vi "3DmenuHandler.vi"(4 "nearClip":sgl, 5 "RawDataFile":path, 6 "farClip":sgl, 7 "FoV":sgl, 10 "ItemTag":string, 11 "3DpicRef":refnum<vi>) -> (0 "error out":errorcluster)   [LabVIEW 2022 SP3]
uses:
  <vilib>/Utility/miscctls.llb/LV3DPointTypeDef.ctl
  <vilib>/Utility/miscctls.llb/LVRectTypeDef.ctl
  <vilib>/Analysis/Matrix/Datatypes/RealMatrix.ctl
  <vilib>/Analysis/baseanly.llb/Matrix Type of Inverse Matrix.ctl
  <vilib>/Analysis/baseanly.llb/Real A x B.vi
  Anemometry/Anemometry Sub Vis/Data_plotting_vis/Results_plotter_Global.vi
  <vilib>/Platform/browser.llb/Open URL in Default Browser (path).vi
  <vilib>/Analysis/baseanly.llb/Real Inverse Matrix.vi
  <vilib>/picture/3D Picture Control/NI_3D Picture Control.lvlib
  <vilib>/Analysis/NI_AALBase.lvlib
  <vilib>/Analysis/Matrix/NI_Matrix.lvlib
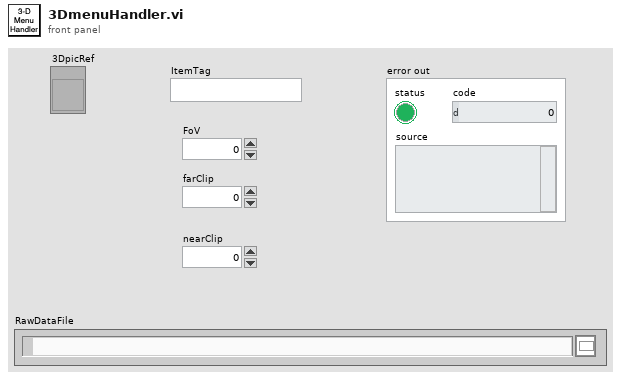
[diagram p1: front panel]
types:
  T1 = enum16{"None", "Spherical", "Flying", "Oriented"}
  T2 = typedef "LV3DPointTypeDef.ctl" = cluster{"X":sgl, "Y":sgl, "Z":sgl}
  T3 = typedef "NI_AALBase.lvlib/Matrix Type of Inverse Matrix.ctl" = enum32{"General", "Positive Definite", "Lower Triangular", "Upper Triangular"}
  T4 = typedef "NI_Matrix.lvlib/RealMatrix.ctl" = dbl[][]
  T5 = enum16{"Open", "Minimized", "Maximized", "Hidden"}
  T6 = typedef "LVRectTypeDef.ctl" = cluster{"Left":i16, "Top":i16, "Right":i16, "Bottom":i16}
  T7 = typedef "imagedata.ctl" = cluster{"image type":i32, "image depth":i32, "image":u8[], "mask":u8[], "colors":u32[], "Rectangle":cluster{"left":i16, "top":i16, "right":i16, "bottom":i16}}
  T8 = typedef "LVRGBAColorTypeDef.ctl" = cluster{"Red":sgl, "Green":sgl, "Blue":sgl, "Alpha":sgl}
  T9 = cluster{"A x B[0]":dbl, "A x B[1]":dbl, "A x B[2]":dbl}
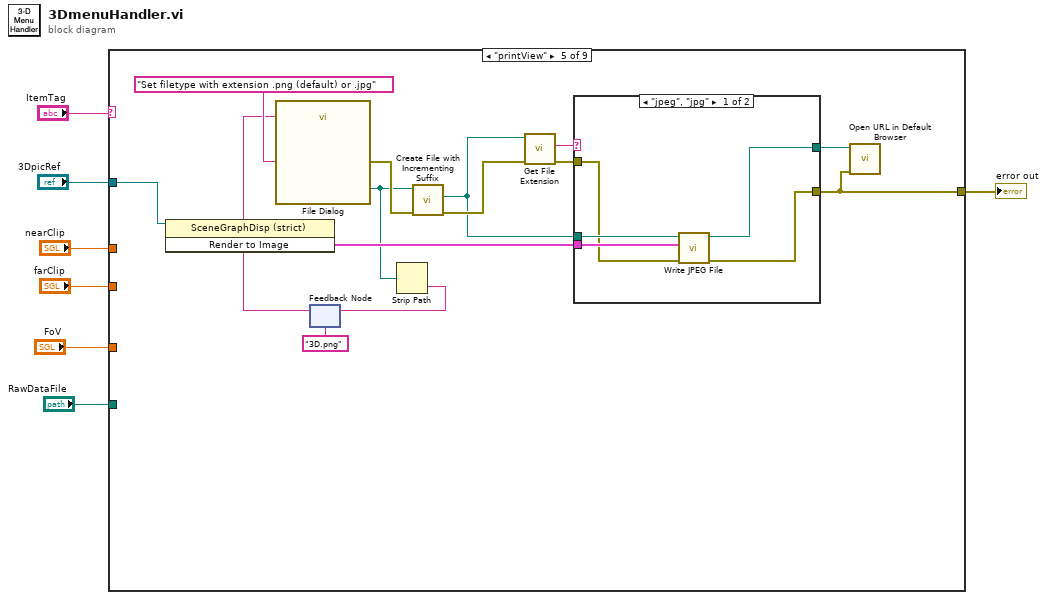
[diagram p0: block diagram]
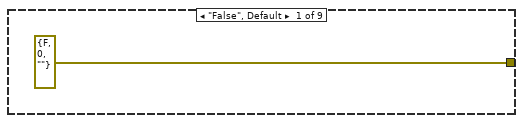
[diagram p2: hidden frame]
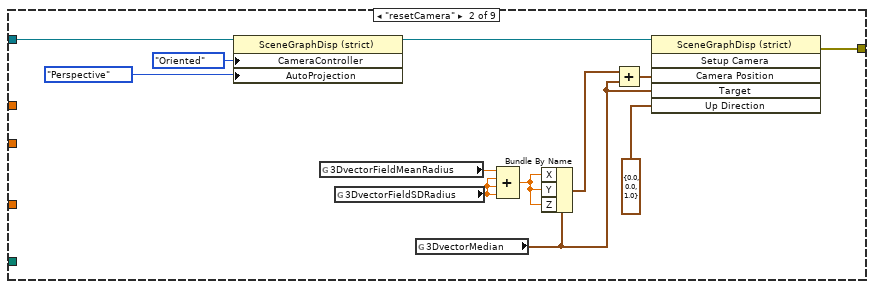
[diagram p3: hidden frame]
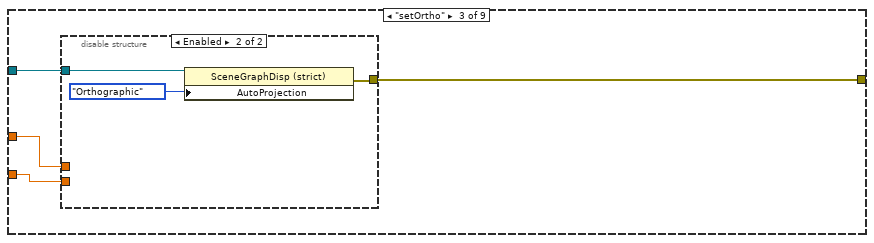
[diagram p4: hidden frame]
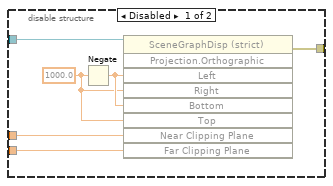
[diagram p5: hidden frame]
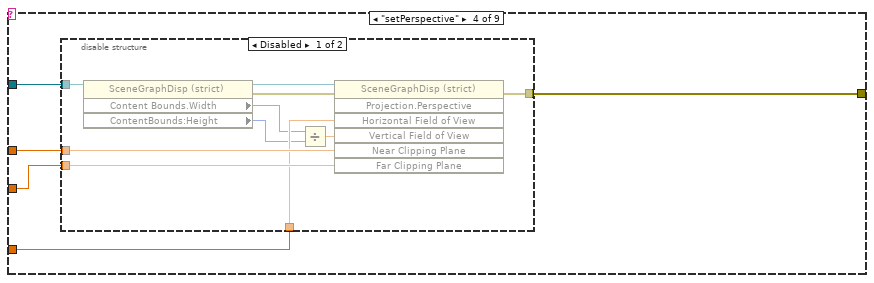
[diagram p6: hidden frame]
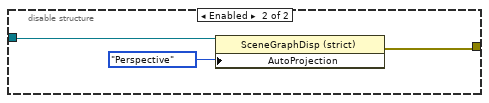
[diagram p7: hidden frame]
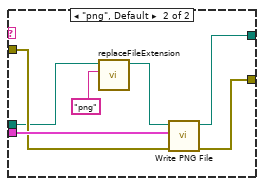
[diagram p8: hidden frame]
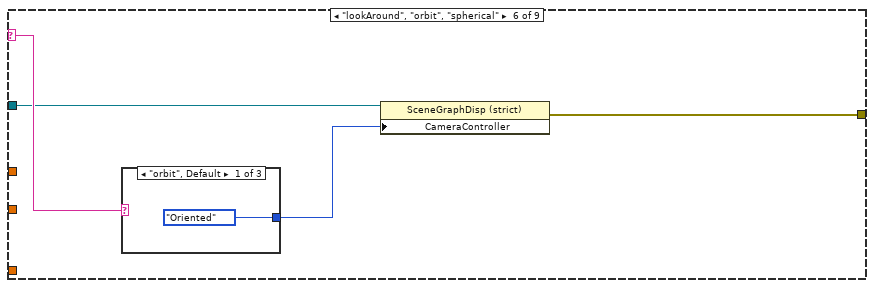
[diagram p9: hidden frame]
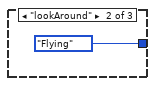
[diagram p10: hidden frame]
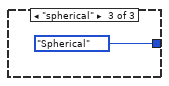
[diagram p11: hidden frame]
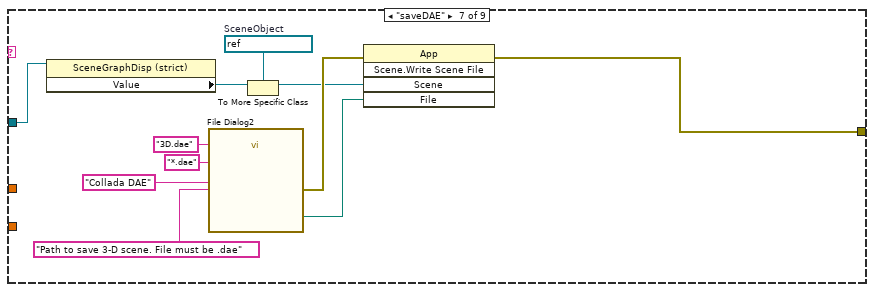
[diagram p12: hidden frame]
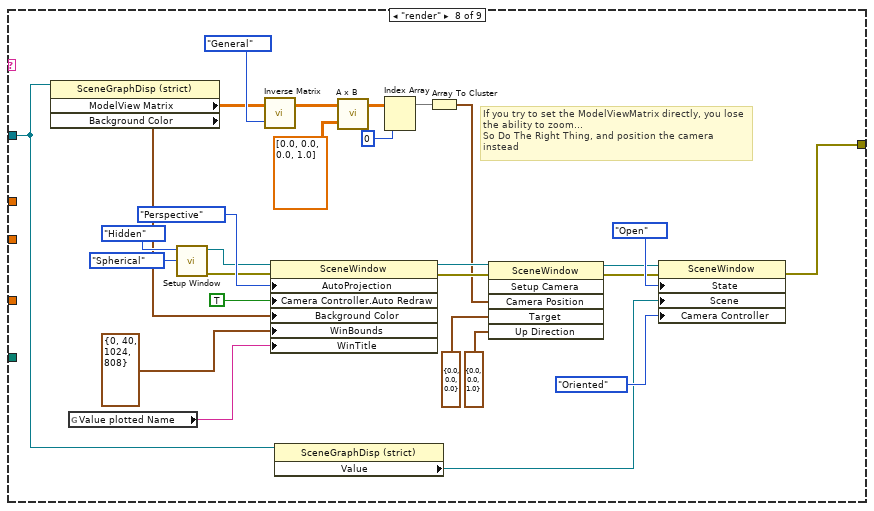
[diagram p13: hidden frame]
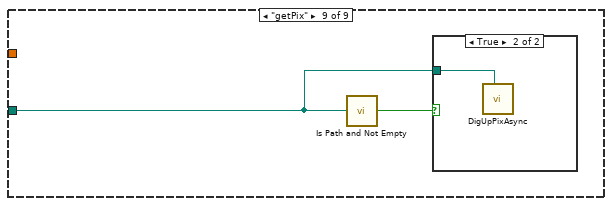
[diagram p14: hidden frame]
diagram:
  n1 = case shown="\"printView\"" "ItemTag" {
    selector: "ItemTag" -> [_ _ _ _ _ w81 _ _ _]
    tunnel: "3DpicRef" -> [_ w14 w21 w34 w62 w80 w87 w98 _]
    tunnel: [errorcluster {"status"=FALSE, "code"=0, "source"=""} ("error out") w10 w24 w38 w60 w79 w88 w99 _] -> w4
    tunnel: "farClip" -> [_ _ w23 w36 _ _ _ _ _]
    tunnel: "nearClip" -> [_ _ w22 w37 _ _ _ _ _]
    tunnel: "FoV" -> [_ _ _ w35 _ _ _ _ _]
    tunnel: "RawDataFile" -> [_ _ _ _ _ _ _ _ w125]
    frame "False", Default {
    }
    frame "resetCamera" {
      n2 = property class="SceneGraphDisp (strict)"(reference=w14, "CameraController"=T1."Oriented" ("Camera Controller:Type"), "AutoProjection"=enum16{"None", "Perspective", "Orthographic"}."Perspective" ("Automatic Projection Mode")) -> (reference out=w13:refnum<vi>)  [unwired: 1 in, 1 out]
      n3 = global read "Results_plotter_Global.vi" "3DvectorFieldMeanRadius"() -> (w19:dbl)
      n4 = global read "Results_plotter_Global.vi" "3DvectorFieldSDRadius"() -> (w9:dbl)
      n5 = global read "Results_plotter_Global.vi" "3DvectorMedian"() -> (w15:cluster{"X":sgl, "Y":sgl, "Z":sgl})
      n6 = Compound Arithmetic op=ADD(w19, w9, w9, w9) -> (w18:dbl)
      n7 = Bundle By Name(cluster=w15, "X"=w18, "Y"=w18, "Z"=w18) -> (w17:cluster{"X":sgl, "Y":sgl, "Z":sgl})
      n8 = Add(x=w17, y=w15) -> (x+y=w16:cluster{"X":sgl, "Y":sgl, "Z":sgl})
      n9 = invoke class="SceneGraphDisp (strict)" method="Setup Camera"(reference=w13, "Camera Position"=w16, "Target"=w15, "Up Direction"=T2 {"X"=0.0, "Y"=0.0, "Z"=1.0}) -> (error out=w10:errorcluster)  [unwired: 2 in, 5 out]
    }
    frame "setOrtho" {
      n10 = disable-structure shown="Enabled" {
        disable-tunnel: [w30 w31] -> w24
        disable-tunnel: w23 -> [w27 _]
        disable-tunnel: w22 -> [w26 _]
        disable-tunnel: w21 -> [w25 w32]
        frame Disabled {
          w28 = sgl 1000.0 ("Left")
          n11 = Negate(x=w28) -> (-x=w29:sgl)
          n12 = invoke class="SceneGraphDisp (strict)" method="Projection.Orthographic"(reference=w25, "Left"=w29, "Right"=w28, "Bottom"=w29, "Top"=w28, "Near Clipping Plane"=w26, "Far Clipping Plane"=w27) -> (error out=w30:errorcluster)  [unwired: 2 in, 8 out]
        }
        frame Enabled {
          n13 = property class="SceneGraphDisp (strict)"(reference=w32, "AutoProjection"=enum16{"None", "Perspective", "Orthographic"}."Orthographic" ("Automatic Projection Mode")) -> (error out=w31:errorcluster)  [unwired: 1 in, 1 out]
        }
      }
    }
    frame "setPerspective" {
      n14 = disable-structure shown="Disabled" {
        disable-tunnel: [w48 w49] -> w38
        disable-tunnel: w37 -> [w47 _]
        disable-tunnel: w36 -> [w46 _]
        disable-tunnel: w35 -> [w45 _]
        disable-tunnel: w34 -> [w44 w50]
        frame Disabled {
          n15 = property class="SceneGraphDisp (strict)"(reference=w44) -> (reference out=w41:refnum<vi>, error out=w39:errorcluster, "Content Bounds.Width"=w43:u32, "ContentBounds:Height"=w42:u32)  [unwired: 1 in]
          n16 = Divide(x=w43, y=w42) -> (x/y=w40:dbl)
          n17 = invoke class="SceneGraphDisp (strict)" method="Projection.Perspective"(reference=w41, error in=w39, "Horizontal Field of View"=w45, "Vertical Field of View"=w40, "Near Clipping Plane"=w47, "Far Clipping Plane"=w46) -> (error out=w48:errorcluster)  [unwired: 1 in, 6 out]
        }
        frame Enabled {
          n18 = property class="SceneGraphDisp (strict)"(reference=w50, "AutoProjection"=enum16{"None", "Perspective", "Orthographic"}."Perspective" ("Automatic Projection Mode")) -> (error out=w49:errorcluster)  [unwired: 1 in, 1 out]
        }
      }
    }
    frame "printView" {
      n19 = invoke on="Invoke Node" class="SceneGraphDisp (strict)" method="Render to Image"(reference=w62) -> ("Get Image"=w65:T7)  [unwired: 2 in, 2 out]
      n20 = feedback #1("3D.png" ("default name")) -> (w52:string)
      n21 = call "File Dialog"("prompt"="Set filetype with extension .png (default) or .jpg", "default name"=w52) -> ("selected path"=w55:path, "error out"=w58:errorcluster)  [unwired: 10 in, 2 out]
      n22 = Strip Path(path=w55) -> (name=w54:string)  [unwired: 1 out]
      n23 = feedback-in #1(w54) -> ()
      n24 = call <vilib>:"Create File with Incrementing Suffix.vi"("error in (no error)"=w58, "file path"=w55) -> ("error out"=w57:errorcluster, "actual path"=w56:path)  [unwired: 7 in, 1 out]
      n25 = call <vilib>:"Get File Extension.vi"("error in (no error)"=w57, "file"=w56) -> ("error out"=w61:errorcluster, "lowercase file extension"=w64:string)  [unwired: 5 in, 3 out]
      n26 = case shown="\"jpeg\", \"jpg\"" w64 {
        tunnel: w65 -> [w69 w77]
        tunnel: w56 -> [w70 w73]
        tunnel: w61 -> [w68 w75]
        tunnel: [w67 w76] -> w60
        tunnel: [w66 w71] -> w59
        frame "jpeg", "jpg" {
          n27 = call <vilib>:"Write JPEG File.vi"("error in (no error)"=w68, "image data"=w69, "path to JPEG file"=w70) -> ("error out"=w67:errorcluster, "path"=w66:path)  [unwired: 7 in]
        }
        frame "png", Default {
          n28 = call "replaceFileExtension.vi"("replacementExtension"="png", "pathIn"=w73) -> ("pathOut"=w72:path)  [unwired: 8 in, 1 out]
          n29 = call <vilib>:"Write PNG File.vi"("error in (no error)"=w75, "image data"=w77, "path to PNG file"=w72) -> ("error out"=w76:errorcluster, "path"=w71:path)  [unwired: 7 in]
        }
      }
      n30 = call-poly <vilib>:"Open URL in Default Browser.vi"("error in (no error)"=w60, "path"=w59) -> ()  [unwired: 4 in, 2 out]
    }
    frame "lookAround", "orbit", "spherical" {
      n31 = case shown="\"orbit\", Default" w81 {
        tunnel: [T1."Oriented" ("Camera Controller:Type") T1."Flying" ("Camera Controller:Type") T1."Spherical" ("Camera Controller:Type")] -> w78
        frame "orbit", Default {
        }
        frame "lookAround" {
        }
        frame "spherical" {
        }
      }
      n32 = property class="SceneGraphDisp (strict)"(reference=w80, "CameraController"=w78) -> (error out=w79:errorcluster)  [unwired: 1 in, 1 out]
    }
    frame "saveDAE" {
      w95 = refnum<vi> refnum  # SceneObject
      n33 = property class="SceneGraphDisp (strict)"(reference=w87) -> ("Value"=w86:refnum<vi>)  [unwired: 1 in, 2 out]
      n34 = call "File Dialog2"("prompt"="Path to save 3-D scene. File must be .dae", "default name"="3D.dae", "pattern (all files)"="*.dae", "pattern label"="Collada DAE") -> ("selected path"=w94:path, "error out"=w89:errorcluster)  [unwired: 8 in, 2 out]
      n35 = To More Specific Class(target class=w95, reference=w86) -> (specific class reference=w85:refnum<vi>)  [unwired: 1 in, 1 out]
      n36 = invoke class="App" method="Scene.Write Scene File"(error in=w89, "Scene"=w85, "File"=w94) -> (error out=w88:errorcluster)  [unwired: 2 in, 4 out]
    }
    frame "render" {
      # "If you try to set the ModelViewMatrix directly, you lose the ability to zoom...\nSo Do The Right Thing, and position the camera instead"
      n37 = property class="SceneGraphDisp (strict)"(reference=w98) -> ("ModelView Matrix"=w101:sgl[][], "Background Color"=w100:T8)  [unwired: 1 in, 2 out]
      n38 = global read "Results_plotter_Global.vi" "Value plotted Name"() -> (w96:string)
      n39 = call <vilib>:"Setup Window.vi"("Camera Controller"=enum16{"None", "Spherical", "Flying"}."Spherical", "Window State"=T5."Hidden") -> ("error out"=w119:errorcluster, "New Window Refnum"=w120:refnum<vi>)  [unwired: 8 in]
      n40 = call-poly <vilib>:"Inverse Matrix.vi"("matrix type"=Matrix_Type_of_Inverse_Matrix."General", "Input Matrix"=w101) -> ("Inverse Matrix"=w109:T4)  [unwired: 1 out]
      n41 = property class="SceneWindow"(reference=w120, error in=w119, "AutoProjection"=enum16{"None", "Perspective", "Orthographic"}."Perspective" ("Automatic Projection Mode"), "Camera Controller.Auto Redraw"=TRUE ("Camera Controller:Auto Redraw"), "Background Color"=w100, "WinBounds"=T6 {"Left"=0, "Top"=40, "Right"=1024, "Bottom"=808} ("Window Bounds"), "WinTitle"=w96) -> (reference out=w114:refnum<vi>, error out=w112:errorcluster)
      n42 = property class="SceneGraphDisp (strict)"(reference=w98) -> ("Value"=w97:refnum<vi>)  [unwired: 1 in, 2 out]
      n43 = call-poly <vilib>:"A x B.vi"("B"=T4 [[0.0], [0.0], [0.0], [1.0]], "A"=w109) -> ("A x B"=w107:T4)  [unwired: 1 out]
      n44 = Index Array(array=w107, index (col)=0 ("disabled index (col)")) -> (element=w106:dbl[])  [unwired: 1 in]
      n45 = Array To Cluster(array=w106) -> (cluster=w104:T9)
      n46 = invoke class="SceneWindow" method="Setup Camera"(reference=w114, error in=w112, "Camera Position"=w104, "Target"=T2 {"X"=0.0, "Y"=0.0, "Z"=0.0}, "Up Direction"=T2 {"X"=0.0, "Y"=0.0, "Z"=1.0}) -> (reference out=w113:refnum<vi>, error out=w111:errorcluster)  [unwired: 1 in, 4 out]
      n47 = property class="SceneWindow"(reference=w113, error in=w111, "State"=T5."Open" ("Window State"), "Scene"=w97, "Camera Controller"=T1."Oriented" ("Camera Controller:Type")) -> (error out=w99:errorcluster)  [unwired: 1 out]
    }
    frame "getPix" {
      n48 = call <vilib>:"Is Path and Not Empty.vi"("path"=w125) -> ("Is Path and Not Empty?"=w124:bool)  [unwired: 4 in]
      n49 = case shown="True" w124 {
        tunnel: w125 -> [_ w126]
        frame False {
        }
        frame True {
          n50 = call "DigUpPixAsync.vi"("File Path"=w126) -> ()  [unwired: 11 in]
        }
      }
    }
  }
  "error out" <- w4
